vi "CalibMatrix (SubVI).vi"(0 "Calibration Files":path[](array[path])) -> (1 "Calib Matrix":dbl[][](array[numeric]), 2 "error out":errorcluster)   [LabVIEW 2011]
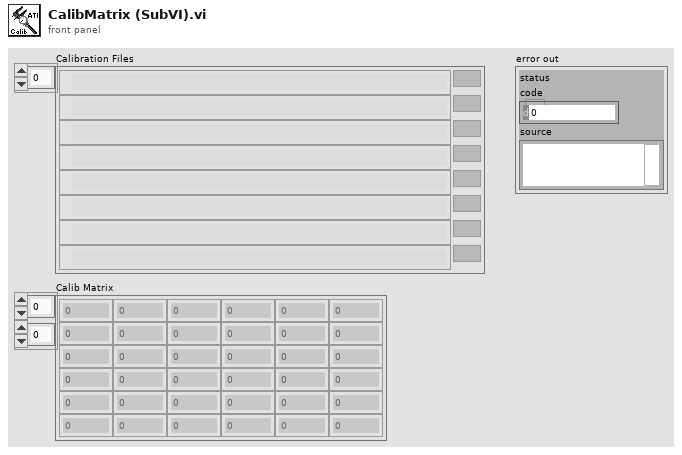
[diagram p1: front panel]
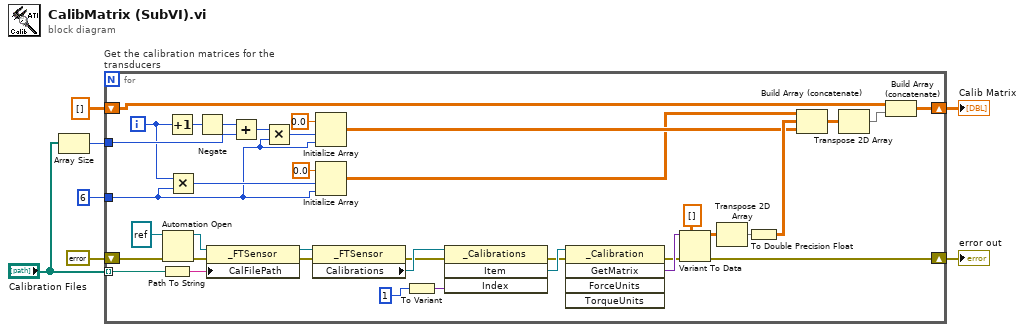
[diagram p0: block diagram]
diagram:
  n1 = Array Size(array="Calibration Files") -> (size(s)=w6:i32)
  n2 = for "Get the calibration matrices for the transducers" {
    tunnel: "Calibration Files" -> [w42] mode=indexing
    shift-right: [w33] -> w1
    shift-left: errorcluster {"status"=FALSE, "code"=0, "source"=""} ("error out") -> [w30]
    tunnel: 6 ("y") -> [w12]
    tunnel: w6 -> [w24]
    shift-right: [w8] -> w7
    shift-left: dbl[][] [] -> [w9]
    i -> [w23]
    n3 = Path To String(path=w42) -> (string=w41:string)
    n4 = Automation Open(error in (no error)=w30, Automation Refnum=refnum<k7> refnum ("ATIDAQFT._FTSensor")) -> (Automation Refnum=w31:refnum<k7>, error out=w29:errorcluster)  [unwired: 1 in, 1 out]
    n5 = Increment(x=w23) -> (x+1=w26:i32)
    n6 = Multiply(x=w23, y=w12) -> (x*y=w14:i32)
    n7 = Negate(x=w26) -> (-x=w25:i32)
    n8 = property class="_FTSensor"(reference=w31, error in=w29, "CalFilePath"=w41) -> (reference out=w43:refnum<k7>, error out=w37:errorcluster)
    n9 = Add(x=w25, y=w24) -> (x+y=w13:i32)
    n10 = Multiply(x=w13, y=w12) -> (x*y=w15:i32)
    n11 = property class="_FTSensor"(reference=w43, error in=w37) -> (error out=w36:errorcluster, "Calibrations"=w44:refnum<k7>)  [unwired: 1 out]
    n12 = Initialize Array(0.0 ("element"), w15, w12) -> (w17:dbl[][])
    n13 = Initialize Array(0.0 ("element"), w14, w12) -> (w16:dbl[][])
    n14 = To Variant(anything=i8 1 ("Index")) -> (Variant=w10:variant)
    n15 = invoke class="_Calibrations" method="Item"(reference=w44, error in=w36, "Index"=w10) -> (error out=w35:errorcluster, "Item"=w40:refnum<k7>)  [unwired: 1 in, 2 out]
    n16 = invoke class="_Calibration" method="GetMatrix"(reference=w40, error in=w35) -> (error out=w34:errorcluster, "GetMatrix"=w39:variant)  [unwired: 3 in, 3 out]
    n17 = Variant To Data(error in=w34, type=sgl[][] [], Variant=w39) -> (data=w22:sgl[][], error out=w33:errorcluster)
    n18 = Transpose 2D Array(2D array=w22) -> (transposed array=w20:sgl[][])
    n19 = To Double Precision Float(number=w20) -> (double precision float=w19:dbl[][])
    n20 = Build Array (concatenate)(w16, w19, w17) -> (w21:dbl[][])
    n21 = Transpose 2D Array(2D array=w21) -> (transposed array=w18:dbl[][])
    n22 = Build Array (concatenate)(w9, w18) -> (w8:dbl[][])
  }
  "Calib Matrix" <- w7
  "error out" <- w1
